vi "ExposeMapperNetObjectToLabviewObj.vi"(11 "Value":variant) -> (3 "variant":variant)   [LabVIEW 2017]
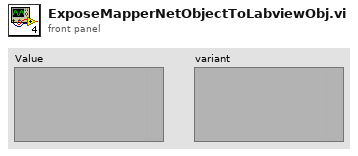
[diagram p1: front panel]
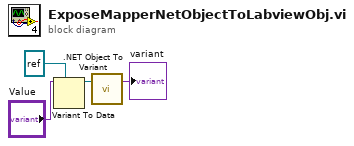
[diagram p0: block diagram]
diagram:
  n1 = Variant To Data(type=refnum<k24> refnum (".NET object"), Variant="Value") -> (data=w3:refnum<k24>)  [unwired: 1 in, 1 out]
  n2 = call <vilib>:".NET Object To Variant.vi"(".NET object"=w3) -> ("variant"=→"variant":variant)  [unwired: 1 in, 1 out]
